vi "cluster_to_array.vi"(11 "Cluster":T1={"Terminal Configuration"=-1, "Min Voltage"=-5.0, "Physical Channel"="Dev1/ai0", "Max Voltage"=5.0, "function"="", "on/off"=FALSE, "物理量"="", "单位"=""} {"Terminal Configuration" items=["default"=-1, "RSE"=10083, "NRSE"=10078, "Differential"=10106, "Pseudodifferential"=12529]}) -> (3 "Array - String":string[](array[string]))   [LabVIEW 2024]
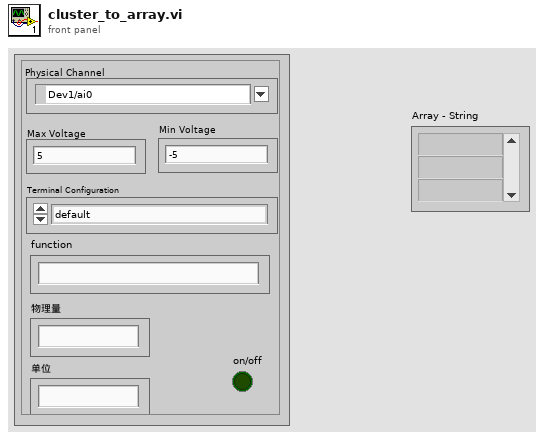
[diagram p1: front panel]
types:
  T1 = cluster{"Terminal Configuration":i32, "Min Voltage":dbl, "Physical Channel":tag, "Max Voltage":dbl, "function":string, "on/off":bool, "物理量":string, "单位":string}
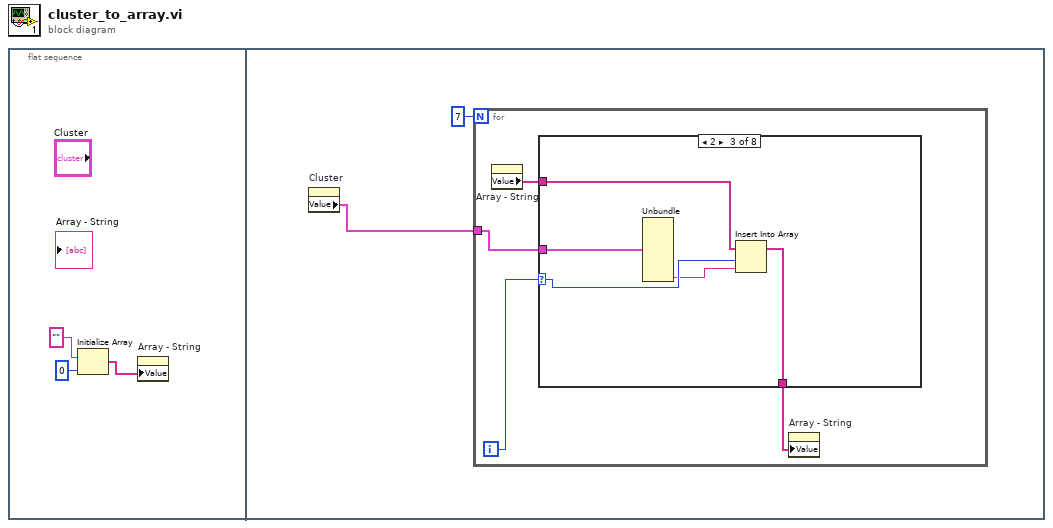
[diagram p0: block diagram]
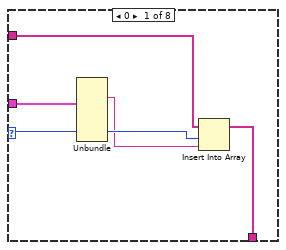
[diagram p2: hidden frame]
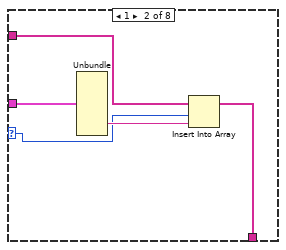
[diagram p3: hidden frame]
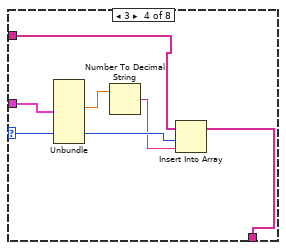
[diagram p4: hidden frame]
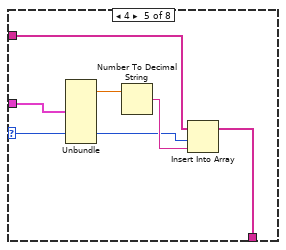
[diagram p5: hidden frame]
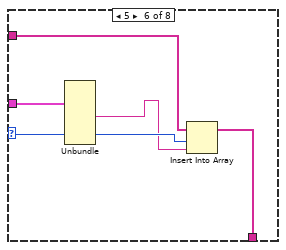
[diagram p6: hidden frame]
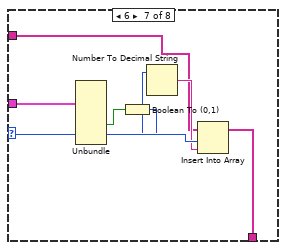
[diagram p7: hidden frame]
diagram:
  n1 = flat-sequence {
    frame #0 {
      n2 = Initialize Array("", 0 ("dimension size")) -> (w1:string[])
      n3 = property on="Array - String" class="Arr (strict)"("Value"=w1) -> ()  [unwired: 2 in, 2 out]
    }
    frame #1 {
      n4 = property on="Cluster" class="Clust (strict)"() -> ("Value"=w4:T1)  [unwired: 2 in, 2 out]
      n5 = for {
        N: 7 -> [_]
        tunnel: w4 -> [w9]
        i -> [w8]
        n6 = property on="Array - String" class="Arr (strict)"() -> ("Value"=w7:string[])  [unwired: 2 in, 2 out]
        n7 = case shown="2" w8 {
          selector: w8 -> [w14 w16 w23 w29 w35 w41 w47 _]
          tunnel: w9 -> [w13 w19 w24 w30 w34 w40 w48 _]
          tunnel: w7 -> [w11 w17 w22 w25 w33 w37 w42 w49]
          tunnel: [w10 w15 w20 w26 w32 w38 w43 w49] -> w6
          frame 0 {
            n8 = Unbundle(w13) -> ("Physical Channel"=w12:tag)  [unwired: 7 out]
            n9 = Insert Into Array(array=w11, index=w14, new element=w12) -> (w10:string[])
          }
          frame 1 {
            n10 = Unbundle(w19) -> ("物理量"=w18:string)  [unwired: 7 out]
            n11 = Insert Into Array(array=w17, index=w16, new element=w18) -> (w15:string[])
          }
          frame 2 {
            n12 = Unbundle(w24) -> ("单位"=w21:string)  [unwired: 7 out]
            n13 = Insert Into Array(array=w22, index=w23, new element=w21) -> (w20:string[])
          }
          frame 3 {
            n14 = Unbundle(w30) -> ("Max Voltage"=w28:dbl)  [unwired: 7 out]
            n15 = Number To Decimal String(number=w28) -> (decimal integer string=w27:string)  [unwired: 1 in]
            n16 = Insert Into Array(array=w25, index=w29, new element=w27) -> (w26:string[])
          }
          frame 4 {
            n17 = Unbundle(w34) -> ("Min Voltage"=w31:dbl)  [unwired: 7 out]
            n18 = Number To Decimal String(number=w31) -> (decimal integer string=w36:string)  [unwired: 1 in]
            n19 = Insert Into Array(array=w33, index=w35, new element=w36) -> (w32:string[])
          }
          frame 5 {
            n20 = Unbundle(w40) -> ("function"=w39:string)  [unwired: 7 out]
            n21 = Insert Into Array(array=w37, index=w41, new element=w39) -> (w38:string[])
          }
          frame 6 {
            n22 = Unbundle(w48) -> ("on/off"=w46:bool)  [unwired: 7 out]
            n23 = Boolean To (0,1)(Boolean=w46) -> (0, 1=w44:i16)
            n24 = Number To Decimal String(number=w44) -> (decimal integer string=w45:string)  [unwired: 1 in]
            n25 = Insert Into Array(array=w42, index=w47, new element=w45) -> (w43:string[])
          }
          frame 7, Default {
          }
        }
        n26 = property on="Array - String" class="Arr (strict)"("Value"=w6) -> ()  [unwired: 2 in, 2 out]
      }
    }
  }
